vi "(SubVI) Delete Length offset of xDNA and Force.vi"(2 "Length offset":dbl, 3 "xDNA cut outside (nm)":dbl=99999.0, 4 "xDNA":dbl[](array[numeric]), 5 "Force":dbl[](array[numeric])) -> (0 "cut-full xDNA":dbl[](array[numeric]), 1 "cut-full Force":dbl[](array[numeric]))   [LabVIEW 2014]
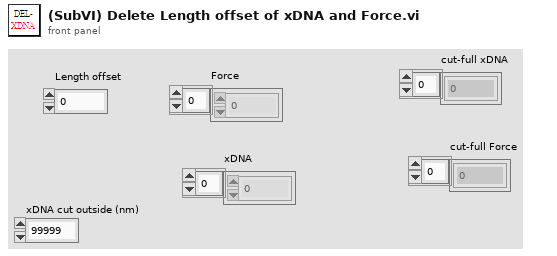
[diagram p1: front panel]
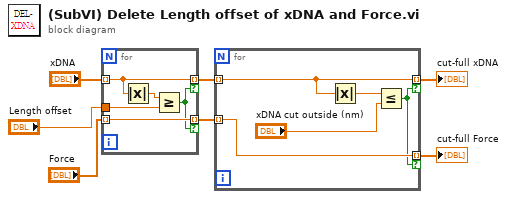
[diagram p0: block diagram]
diagram:
  n1 = for {
    tunnel: "xDNA" -> [w11] mode=indexing
    tunnel: [w11] -> w4 mode=indexing if=w8
    tunnel: "Force" -> [w12] mode=indexing
    tunnel: [w12] -> w3 mode=indexing if=w8
    tunnel: "Length offset" -> [w9]
    n2 = Absolute Value(x=w11) -> (abs(x)=w10:dbl)
    n3 = Greater Or Equal?(x=w10, y=w9) -> (x >= y?=w8:bool)
  }
  n4 = for {
    tunnel: [w14] -> w2 mode=indexing if=w15
    tunnel: w4 -> [w14] mode=indexing
    tunnel: w3 -> [w17] mode=indexing
    tunnel: [w17] -> w1 mode=indexing if=w15
    n5 = Absolute Value(x=w14) -> (abs(x)=w13:dbl)
    n6 = Less Or Equal?(x=w13, y="xDNA cut outside (nm)") -> (x <= y?=w15:bool)
  }
  "cut-full Force" <- w1
  "cut-full xDNA" <- w2
